vi "SRV_VIG_Streaming States.vi"(7 "Streaming States":T1, 12 "Method (Get)":enum16{"Get", "Set"}(ring)) -> (8 "Streaming States out":T1)   [LabVIEW 2009]
uses:
  SRV_Streaming States.ctl
  SRV_Streaming State.ctl
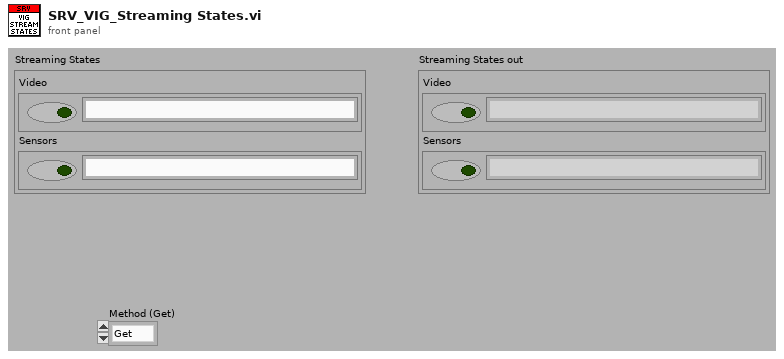
[diagram p1: front panel]
types:
  T1 = typedef "SRV_Streaming States.ctl" = cluster{"Video":T2, "Sensors":T2}
  T2 = typedef "SRV_Streaming State.ctl" = cluster{"Enabled":bool, "Data":string}
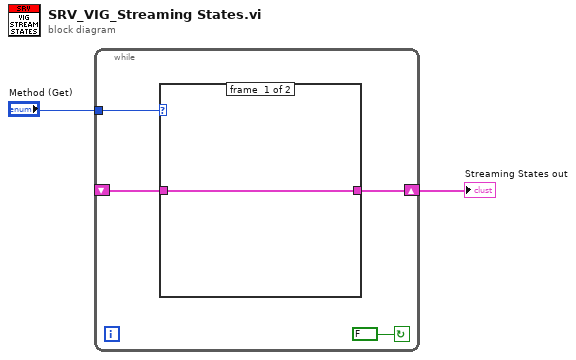
[diagram p0: block diagram]
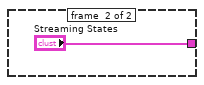
[diagram p2: hidden frame]
diagram:
  n1 = while {
    shift-right: [w4] -> w1
    shift-left: _ -> [w3]
    tunnel: "Method (Get)" -> [w5]
    stop <- FALSE continue-if-true
    n2 = case shown="\"Set\"" w5 {
      tunnel: [w7 "Streaming States"] -> w4
      tunnel: w3 -> [w7 _]
      frame #0 {
      }
      frame #1 {
      }
    }
  }
  "Streaming States out" <- w1
